vi "libssh2_channel_request_pty_ex.vi"(4 "height_px":i32, 5 "height":i32=24, 6 "width_px":i32, 7 "width":i32=80, 8 "error in (no error)":errorcluster, 9 "modes":string, 10 "term":string, 11 "channel":T1) -> (0 "error out":errorcluster)   [LabVIEW 2013, in "libssh2.lvlib"]
doc: "Request a pseudo-terminal on a channel."
uses:
  libssh2.lvlib
  Channel Refnum.ctl
  Not A Channel.vi
  <vilib>/Utility/error.llb/Error Cluster From Error Code.vi
  Global Settings.vi
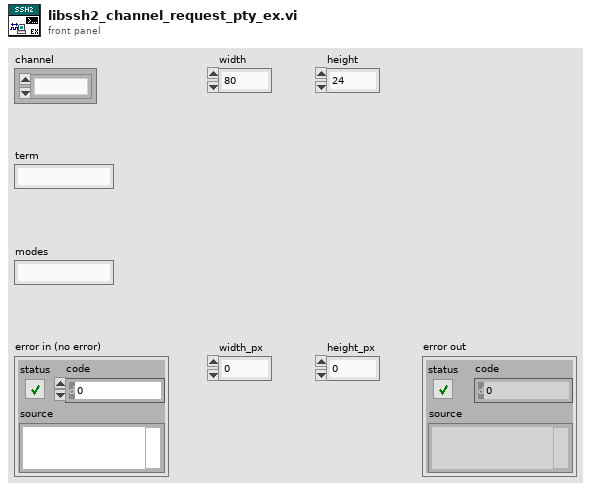
[diagram p1: front panel]
types:
  T1 = typedef "libssh2.lvlib/Channel Refnum.ctl" = refnum<k1>
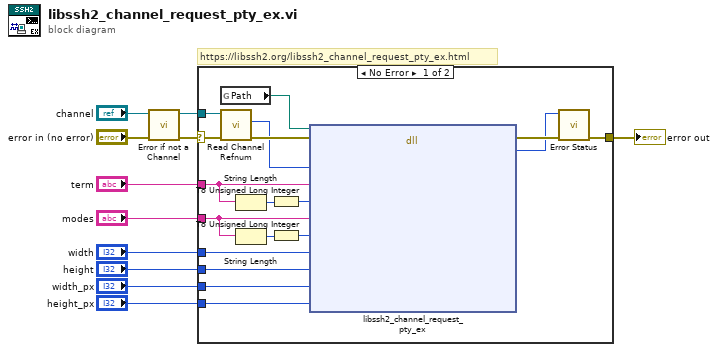
[diagram p0: block diagram]
diagram:
  # "https://libssh2.org/libssh2_channel_request_pty_ex.html"
  n1 = call "Error if not a Channel.vi"("error in (no error)"="error in (no error)", "channel"="channel") -> ("error out"=w9:errorcluster, "channel out"=w7:T1)  [unwired: 8 in]
  n2 = case shown="No Error" w9 {
    selector: w9 -> [w29 w30]
    tunnel: [w28 w30] -> w11
    tunnel: w7 -> [w27 _]
    tunnel: "term" -> [w12 _]
    tunnel: "modes" -> [w16 _]
    tunnel: "width" -> [w21 _]
    tunnel: "height" -> [w20 _]
    tunnel: "width_px" -> [w19 _]
    tunnel: "height_px" -> [w18 _]
    frame No Error {
      n3 = global read "Global Settings.vi" "Path"() -> (w23:path)
      n4 = call "Read Channel Refnum.vi"("error in (no error)"=w29, "channel"=w27) -> ("error out"=w25:errorcluster, "LIBSSH2_CHANNEL*"=w24:u64)  [unwired: 8 in]
      n5 = String Length(string=w12) -> (length=w14:i32)
      n6 = String Length(string=w16) -> (length=w17:i32)
      n7 = To Unsigned Long Integer(number=w14) -> (unsigned 32bit integer=w13:u32)
      n8 = To Unsigned Long Integer(number=w17) -> (unsigned 32bit integer=w15:u32)
      n9 = dll-call lib="?" fn="libssh2_channel_request_pty_ex"(path in=w23, error in=w25, "channel"=w24, "term"=w12, "term_len"=w13, "modes"=w16, "modes_len"=w15, "width"=w21, "height"=w20, "width_px"=w19, "height_px"=w18) -> (error out=w26:errorcluster, "return value"=w22:i32)  [unwired: 10 in, 1 out]
      n10 = call "Error Status.vi"("error in (no error)"=w26, "return value"=w22) -> ("error out"=w28:errorcluster)  [unwired: 8 in, 1 out]
    }
    frame Error {
    }
  }
  "error out" <- w11
